vi "pause2.vi"() -> ()   [LabVIEW 2020]
panel:
  in  "pause2":bool
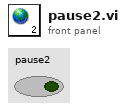
[diagram p1: front panel]
diagram:
